vi "AuMT8852B Request Supported Features From EUT.vi"(8 "error in (no error)":errorcluster, 11 "VISA session":refnum<visa-resource-name>) -> (0 "error out":errorcluster, 2 "error code":i32, 3 "VISA session out":refnum<visa-resource-name>)   [LabVIEW 2017]
doc: "Anritsu MT8852B Bluetooth Tester\n\nRequests the supported features from the EUT whether or not it is already available from a previous request or connection. The features are then available to be read over the GPIB using the SYSCFG? EUTFEAT command (EUT Supported Features Query)."
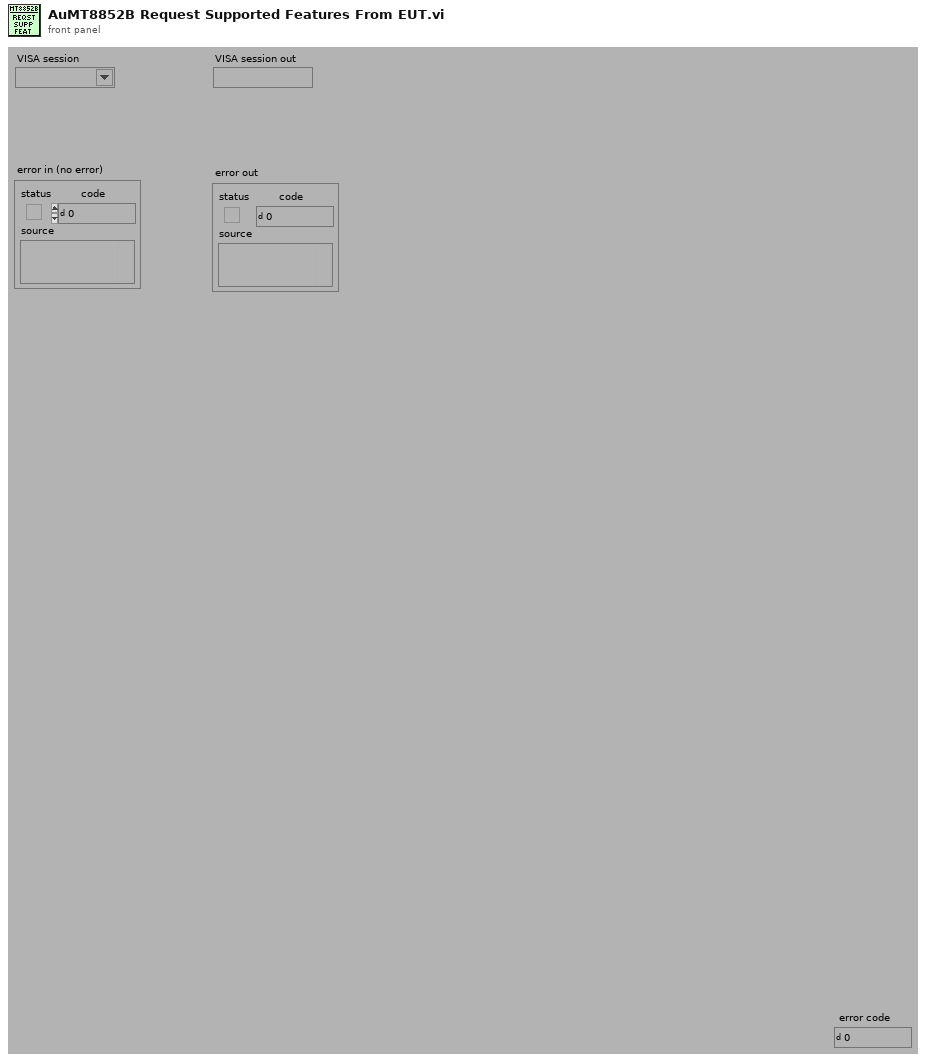
[diagram p1: front panel]
types:
  T1 = enum16{"Simulate", "Range check", "Cache", "Query instrument status"}
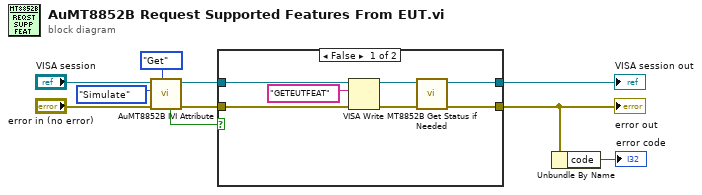
[diagram p0: block diagram]
diagram:
  n1 = call <instrlib>:"AuMT8852B IVI Attribute.vi"("Set/Get (Set)"=enum16{"Set", "Get"}."Get", "error in (no error)"="error in (no error)", "Flag (Simulate)"=T1."Simulate", "VISA session"="VISA session") -> ("error out"=w7:errorcluster, "VISA session out"=w9:refnum<visa-resource-name>, "Value out"=w3:bool)  [unwired: 5 in]
  n2 = case shown="False" w3 {
    tunnel: [w14 w19] -> w10
    tunnel: [w13 w18] -> w1
    tunnel: w9 -> [w16 w19]
    tunnel: w7 -> [w15 w18]
    frame False {
      n3 = VISA Write(VISA resource name=w16, write buffer="GETEUTFEAT" ("write buffer (\"\")"), error in (no error)=w15) -> (VISA resource name out=w11:refnum<visa-resource-name>, error out=w12:errorcluster)  [unwired: 1 out]
      n4 = call <instrlib>:"MT8852B Get Status if Needed.vi"("error in (no error)"=w12, "VISA session"=w11) -> ("error out"=w13:errorcluster, "VISA session out"=w14:refnum<visa-resource-name>)  [unwired: 8 in]
    }
    frame True {
      (unwired) u8 0
    }
  }
  "error out" <- w1
  "VISA session out" <- w10
  n5 = Unbundle By Name(w1) -> ("code"=→"error code":i32)
